vi "Read Density.vi"(8 "error in (no error)":errorcluster, 11 "Bronkhorst Settings in":T1) -> (0 "error out":errorcluster, 1 "Connection Error":bool, 2 "Density kg/m^3":sgl, 3 "Bronkhorst Settings out":T1)   [LabVIEW 2018, in "Bronkhorst M14 Flow Meter.lvlib"]
uses:
  Bronkhorst M14 Flow Meter.lvlib
  Bronkhorst M13 Flow Meter/Settings Cluster.ctl
  <vilib>/regexp/Match Regular Expression.xnode
  <vilib>/ptbypt/NI_PtbyPt.lvlib
  Bronkhorst M13 Flow Meter/Bronkhorst M13 Flow Meter.lvlib
panel:
  out "submatch 1":string
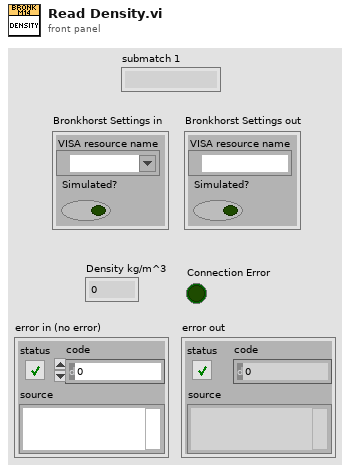
[diagram p1: front panel]
types:
  T1 = typedef "Bronkhorst M13 Flow Meter.lvlib/Settings Cluster.ctl" = cluster{"VISA resource name":refnum<visa-resource-name>, "Simulated?":bool}
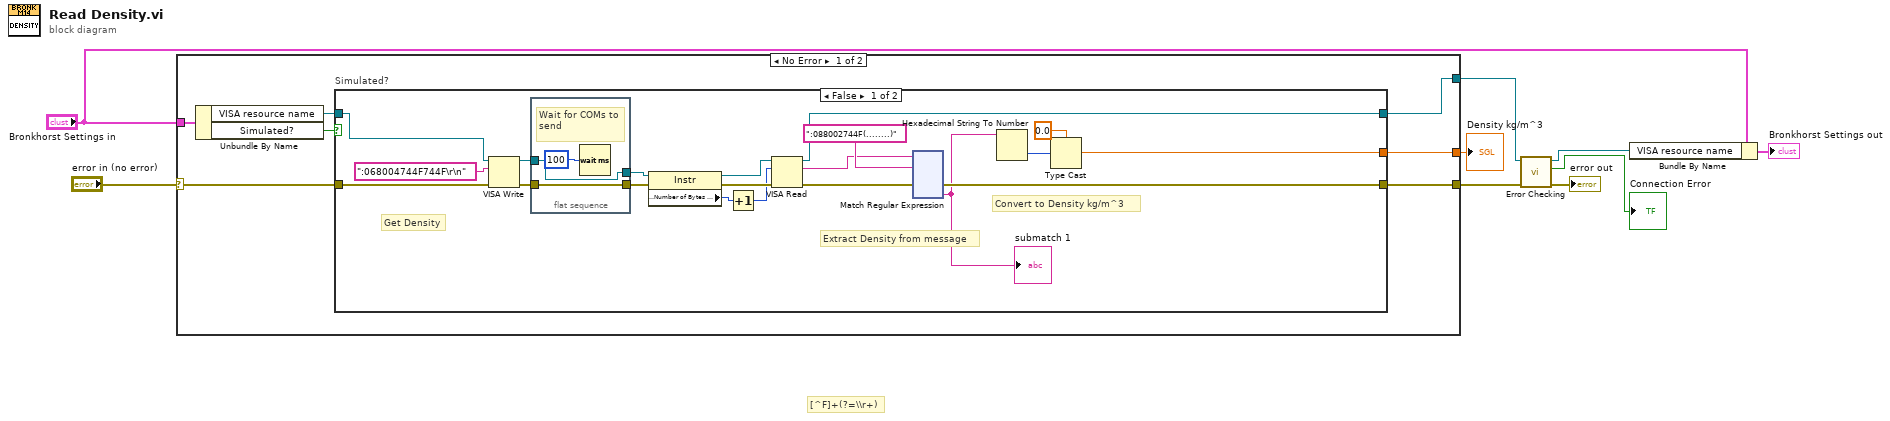
[diagram p0: block diagram]
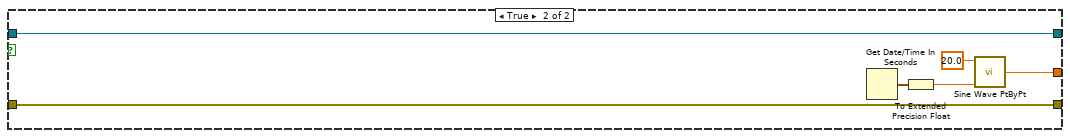
[diagram p2: hidden frame]
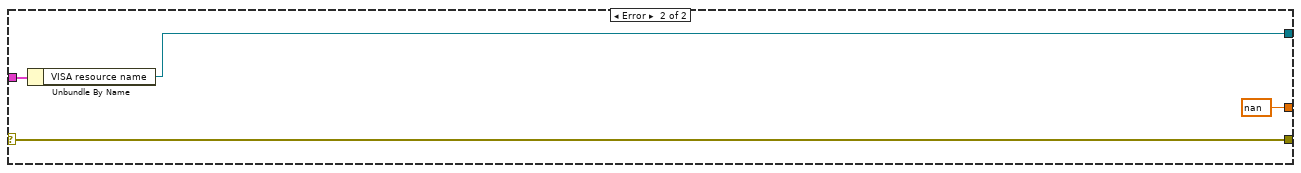
[diagram p3: hidden frame]
diagram:
  # "[^F]+(?=\\\\r+)"
  n1 = case shown="No Error" "error in (no error)" {
    selector: "error in (no error)" -> [w15 w165]
    tunnel: [w14 w165] -> w4
    tunnel: "Bronkhorst Settings in" -> [w13 w164]
    tunnel: [w11 w163] -> w6
    tunnel: [w10 nan ("sine wave")] -> w1
    frame No Error {
      n2 = Unbundle By Name(w13) -> ("VISA resource name"=w12:refnum<visa-resource-name>, "Simulated?"=w16:bool)
      n3 = case "Simulated?" shown="False" w16 {
        tunnel: [w18 w161] -> w14
        tunnel: w15 -> [w28 w161]
        tunnel: [w25 w157] -> w11
        tunnel: w12 -> [w29 w157]
        tunnel: [w22 w156] -> w10
        frame False {
          # "Extract Density from message"
          # "Get Density"
          # "Convert to Density kg/m^3"
          n4 = VISA Write(VISA resource name=w29, write buffer=":068004744F744F\r\n" ("Command"), error in (no error)=w28) -> (VISA resource name out=w33:refnum<visa-resource-name>, error out=w31:errorcluster)  [unwired: 1 out]
          n5 = flat-sequence {
            tunnel: [w155] -> w32
            tunnel: w33 -> [w155]
            tunnel: [w154] -> w30
            tunnel: w31 -> [w154]
            frame #0 {
              # "Wait for COMs to send"
              n6 = Wait (ms)(milliseconds to wait=u32 100) -> ()  [unwired: 1 out]
            }
          }
          n7 = property class="Instr"(reference=w32, error in=w30) -> (reference out=w35:refnum<visa-resource-name>, error out=w34:errorcluster, "Serial Settings:Number of Bytes at Serial Port"=w27:u32)
          n8 = Increment(x=w27) -> (x+1=w26:u32)
          n9 = VISA Read(VISA resource name=w35, byte count=w26, error in (no error)=w34) -> (VISA resource name out=w25:refnum<visa-resource-name>, read buffer=w20:string, error out=w19:errorcluster)  [unwired: 1 out]
          n10 = xnode "Match Regular Expression"("input string"=w20, "regular expression"=":088002744F(........)" ("Regular Expression for Extracting Weight"), "error in"=w19) -> ("error out"=w18:errorcluster, "submatch 1"=w17:string)  [unwired: 3 in, 4 out]
          "submatch 1" <- w17
          n11 = Hexadecimal String To Number(string=w17) -> (number=w23:u32)  [unwired: 2 in, 1 out]
          n12 = Type Cast(type=sgl 0.0, x=w23) -> (*(type *) &x=w22:sgl)
        }
        frame True {
          n13 = Get Date/Time In Seconds() -> (seconds since 1Jan1904=w160:timestamp)
          n14 = To Extended Precision Float(1:w160) -> (0:w159:ext)
          n15 = call <vilib>:"Sine Wave PtByPt.vi"("time"=w159, "amplitude"=20.0) -> ("sine wave"=w156:dbl)  [unwired: 2 in]
        }
      }
    }
    frame Error {
      n16 = Unbundle By Name(w164) -> ("VISA resource name"=w163:refnum<visa-resource-name>)
    }
  }
  "Density kg/m^3" <- w1
  n17 = call "Error Checking.vi"("error in (no error)"=w4, "VISA resource name"=w6) -> ("error out"=→"error out":errorcluster, "Connection Error"=→"Connection Error":bool, "VISA resource name"=w5:refnum<visa-resource-name>)  [unwired: 7 in]
  n18 = Bundle By Name(cluster="Bronkhorst Settings in", "VISA resource name"=w5) -> (→"Bronkhorst Settings out":T1)
